vi "Configure WatchDog (Com).vi"(0 "VISA resource name":refnum<visa-resource-name>, 1 "Value At Timer Expired (1: Last Value)":u16(ring)=1 items=["Preset Value", "Last Value"], 5 "Channel (001)":string="001", 7 "Enable Watchdog Timer (False)":bool, 9 "Timer (30Sec.)":i32=30 min=1 max=120, 11 "error in (no error)":errorcluster) -> (4 "VISA resource name out":refnum<visa-resource-name>, 6 "Channel":string, 15 "error out":errorcluster)   [LabVIEW 2020, in "Yokogawa GX Series.lvlib"]
doc: "Sets the watchdog timer of a communication channel.\n\nCommands: SWDCom"
uses:
  <instrlib>/Yokogawa GX Series/Yokogawa GX Series.lvlib
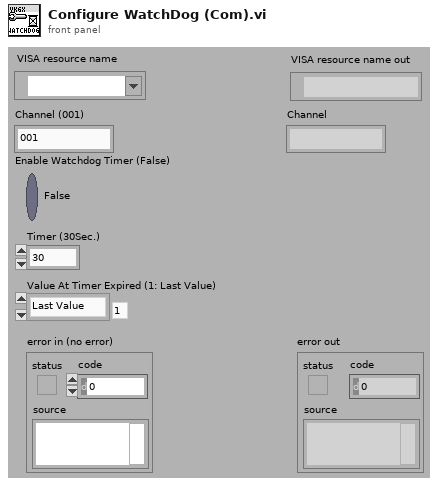
[diagram p1: front panel]
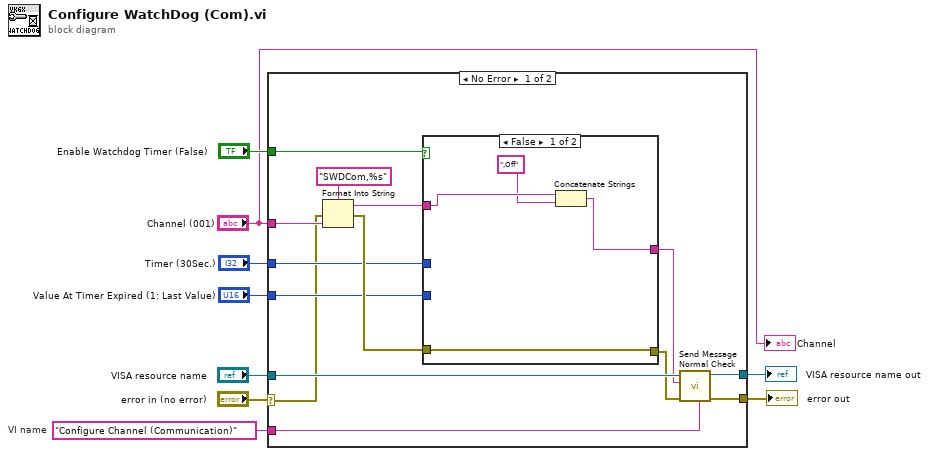
[diagram p0: block diagram]
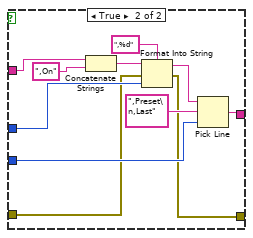
[diagram p2: hidden frame]
diagram:
  w6 = "Configure Channel (Communication)"  # VI name
  n1 = case shown="No Error" "error in (no error)" {
    selector: "error in (no error)" -> [w10 w39]
    tunnel: [w21 w39] -> w9
    tunnel: [w20 w40] -> w8
    tunnel: "VISA resource name" -> [w19 w40]
    tunnel: w6 -> [w18 _]
    tunnel: "Enable Watchdog Timer (False)" -> [w16 _]
    tunnel: "Channel (001)" -> [w15 _]
    tunnel: "Timer (30Sec.)" -> [w14 _]
    tunnel: "Value At Timer Expired (1: Last Value)" -> [w13 _]
    frame No Error {
      n2 = Format Into String(format string="SWDCom,%s", error in=w10, w15) -> (resulting string=w17:string, error out=w22:errorcluster)  [unwired: 1 in]
      n3 = case shown="False" w16 {
        tunnel: w22 -> [w24 w30]
        tunnel: [w24 w28] -> w12
        tunnel: [w25 w29] -> w11
        tunnel: w17 -> [w27 w38]
        tunnel: w14 -> [_ w35]
        tunnel: w13 -> [_ w33]
        frame False {
          n4 = Concatenate Strings(w27, ",Off") -> (w25:string)
        }
        frame True {
          n5 = Concatenate Strings(w38, ",On") -> (w34:string)
          n6 = Format Into String(format string=",%d", initial string=w34, error in=w30, w35) -> (resulting string=w31:string, error out=w28:errorcluster)
          n7 = Pick Line(string ("")=w31, multi-line string=",Preset\n,Last", line index=w33) -> (output string=w29:string)
        }
      }
      n8 = call <instrlib>:"Send Message Normal Check.vi"("Source (\"\")"=w18, "error in (no error)"=w12, "Send Message (\"\")"=w11, "VISA resource name"=w19) -> ("error out"=w21:errorcluster, "VISA resource name out"=w20:refnum<visa-resource-name>)  [unwired: 2 in, 4 out]
    }
    frame Error {
    }
  }
  "error out" <- w9
  "VISA resource name out" <- w8
  "Channel" <- "Channel (001)"
